vi "AddTest.vi"(8 "error in (no error)":errorcluster, 10 "Test":refnum<class "Test.lvclass">, 11 "TestSuite in":refnum<class "TestSuite.lvclass">) -> (0 "error out":errorcluster, 3 "TestSuite out":refnum<class "TestSuite.lvclass">)   [LabVIEW 2017, in "TestSuite.lvclass"]
doc: "Adds a test to the suite."
uses:
  TestSuite.lvclass
  Test/Test.lvclass
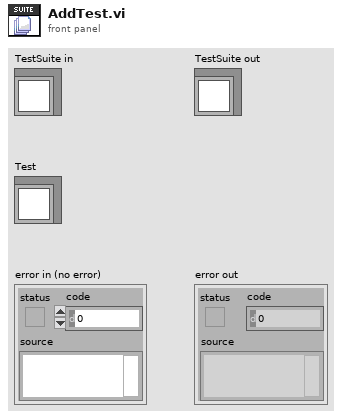
[diagram p1: front panel]
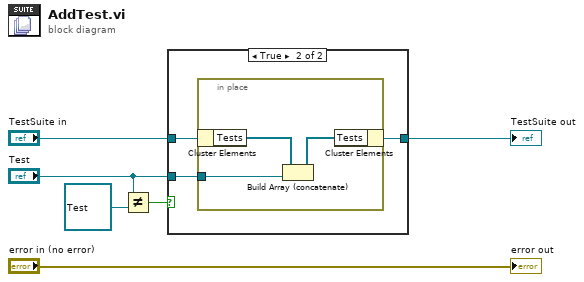
[diagram p0: block diagram]
diagram:
  n1 = Not Equal?(x="Test", y=refnum<class "Test.lvclass"> refnum) -> (x != y?=w1:bool)
  n2 = case shown="True" w1 {
    tunnel: "TestSuite in" -> [w7 w10]
    tunnel: [w7 w9] -> w4
    tunnel: "Test" -> [_ w8]
    frame False {
    }
    frame True {
      n3 = in-place {
        in-place-border: w8 -> [w11]
        n4 = in-place-cluster #1(w10) -> ("Tests"=w13:refnum<class "Test.lvclass">[])
        n5 = Build Array (concatenate)(w13, w11) -> (w12:refnum<class "Test.lvclass">[])
        n6 = in-place-cluster #1("Tests"=w12) -> (w9:refnum<class "TestSuite.lvclass">)
      }
    }
  }
  "TestSuite out" <- w4
  "error out" <- "error in (no error)"
